vi "终极版程序.vi"() -> ()   [LabVIEW 2013]
uses:
  <vilib>/Platform/TimedLoop/XDataNode/timing_clust.ctl
  <vilib>/Platform/TimedLoop/XDataNode/nitl_modes.ctl
  <vilib>/Platform/TimedLoop/XDataNode/wakeup.ctl
  <vilib>/Simulation/Scripting/Companion Diagram/SimConfigNode/SimParams.ctl
  <vilib>/Simulation/Scripting/Companion Diagram/SimConfigNode/_simSolvers.ctl
  <vilib>/Simulation/Implementation/Shared/SIMSCR Execution Mode.ctl
  <vilib>/Simulation/Param Hierarchy/Typedefs/SIMPH Param Control Actions.ctl
  <vilib>/Simulation/Implementation/Shared/SIM limit type.ctl
  <vilib>/Simulation/Implementation/Shared/NILVSim_ParamChanged.vi
  <vilib>/Simulation/Implementation/Shared/NILVSIM_BeginStep.vi
  <vilib>/Simulation/DataSources/Implementation/NILVSim Signal Generator.llb/SIM Signal Generator (scalar).vi
  <vilib>/Simulation/SignalDisplay/Implementation/NILVSim Time Waveform.llb/SIM Time Waveform (vector).vi
  <vilib>/Simulation/SignalArithmetic/Implementation/NILVSim Gain.llb/SIM Gain (scalar).vi
  <vilib>/Simulation/ContinuousLinear/Implementation/NILVSim Integrator new.llb/SIM Integrator distributor (scalar).vi
  <vilib>/Simulation/Nonlinear/Implementation/NILVSim Saturation.llb/SIM Saturation (scalar).vi
  <vilib>/Simulation/SignalDisplay/Implementation/NILVSim Time Waveform.llb/SIM Time Waveform (scalar).vi
  <vilib>/Simulation/Utility/Implementation/NILVSim Memory.llb/NILVSim Memory (core).vi
  <vilib>/Simulation/ContinuousLinear/Implementation/NILVSim Integrator new.llb/SIM Integrator collector (scalar).vi
  <vilib>/Simulation/Implementation/Shared/NILVSim_Manager.vi
  <vilib>/Simulation/Implementation/Shared/NILVSim_FinalizeModel.vi
  <vilib>/Simulation/Implementation/Shared/SIM Unbundle Sim Info.vi
  <vilib>/Utility/error.llb/Clear Errors.vi
  <vilib>/Simulation/Implementation/Shared/NILVSim_GetModelError.vi
  <vilib>/Simulation/Implementation/Shared/SIM Bundle Sim Info.vi
  <vilib>/Simulation/Implementation/Shared/SIMSH Read Queue.vi
  <vilib>/Simulation/Implementation/Shared/NILVSim_Initialize.vi
  <vilib>/Simulation/Utility/Implementation/NILVSim Get Time and IsAcceptedStep.vi
  <vilib>/Platform/TimedLoop/XDataNode/XDataNode.xnode
  <vilib>/Simulation/Scripting/Companion Diagram/SimConfigNode/SimDog.xnode
  <vilib>/Simulation/Implementation/XNodeFramework/SimXNode/SimX.xnode
  <vilib>/Platform/TimedLoop/XDataNode/XDNodeRunTimeDep.lvlib
  <vilib>/Simulation/ContinuousLinear/Implementation/NILVSim Integrator new.llb/SIM Integrator (scalar).vi
  <vilib>/Simulation/Implementation/Shared/NI_SIM_Implementation.lvlib
panel:
  in  "信号发生器":T1
  out "速度（rad/s）":waveform(dbl)[](graph)
  out "电压（V）":waveform(dbl)(graph)
  in  "PID控制参数":cluster{"kp":dbl, "bsp":dbl, "ki":dbl}
  out "Instrument":string="If you want to exit program,Please press \"Exit Program\" button"
  out "AxMaxVel":bool
  out "DeviceNum List":u32[](array[numeric])
  out "Servo_Off":bool
  in  "Servo_On":bool
  in  "Servo On":bool
  in  "Clear":bool
  out "ChangeV Success":bool
  in  "ChangeV":bool
  in  "Change Velocity":dbl=10000.0
  out "Axis State:":string
  out "CloseSuccess":bool
  in  "Device Type":u16(ring) items=["PCI-1240 (M0)"]
  out "PAR_AxVelHigh":dbl=500.0
  out "Ret_GetCommandPosition":u32
  out "Exit Program":bool
  out "DeviceOpened":bool
  out "AxisOpened":bool
  out "AxisHandle_Array":u32[](array[numeric])
  out "DevAxesCount":u32
  out "EmgSucces":bool
  out "DecSuccess":bool
  in  "Stop Mode":enum32{"Dec", "Emg"}(radio)
  out "RelSucces":bool
  in  "Distance":dbl=50000.0
  out "AbsSuccess":bool
  in  "Movement Mode":enum32{"Absolute", "Relative"}(radio)=enum."Relative"
  in  "Operate Axis":T2(radio)
  in  "Stop":bool
  in  "Move":bool
  out "ResetCounter":bool
  in  "Reset Counter":bool
  out "Axis Position":T3
  out "DeviceHandle":u32
  in  "Stop":bool
  in  "Close Board":bool
  in  "Open Board":bool
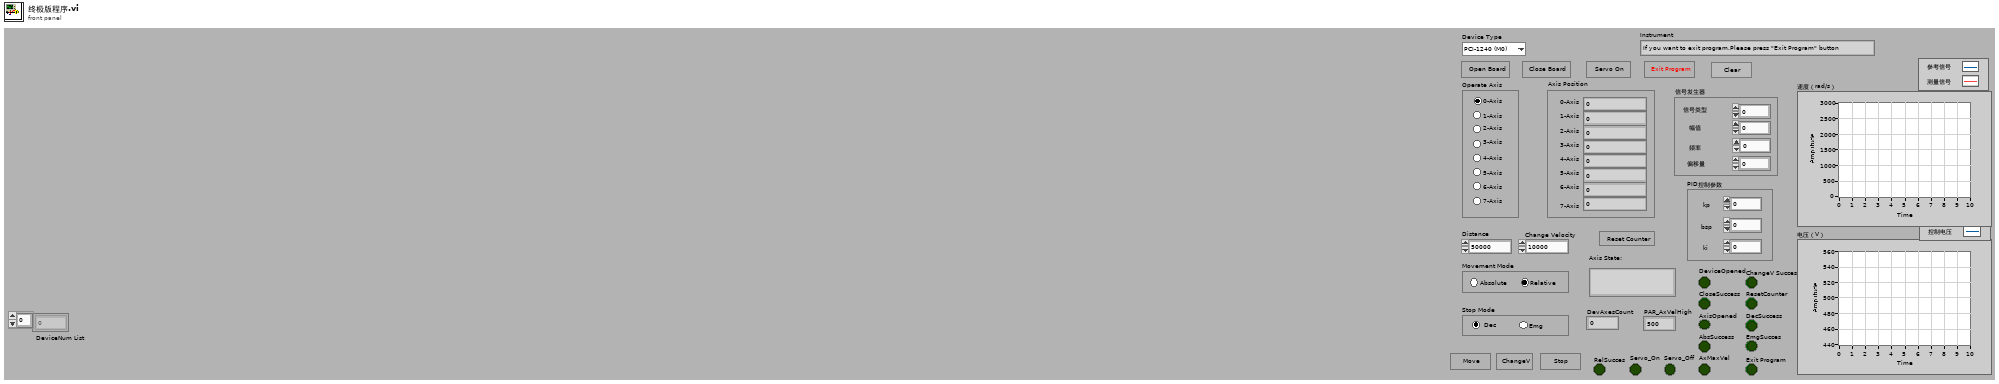
[diagram p1: front panel]
types:
  T1 = cluster{"信号类型":dbl, "幅值":dbl, "频率":dbl, "偏移量":dbl}
  T2 = enum32{"0-Axis", "1-Axis", "2-Axis", "3-Axis", "4-Axis", "5-Axis", "6-Axis", "7-Axis"}
  T3 = cluster{"0-Axis":dbl, "1-Axis":dbl, "2-Axis":dbl, "3-Axis":dbl, "4-Axis":dbl, "5-Axis":dbl, "6-Axis":dbl, "7-Axis":dbl}
  T4 = cluster{"DeviceNum":u32, "U*8 Array":cluster{"U*8 Array[0]":u8, "U*8 Array[1]":u8, "U*8 Array[2]":u8, "U*8 Array[3]":u8, "U*8 Array[4]":u8, "U*8 Array[5]":u8, "U*8 Array[6]":u8, "U*8 Array[7]":u8, "U*8 Array[8]":u8, "U*8 Array[9]":u8, "U*8 Array[10]":u8, "U*8 Array[11]":u8, "U*8 Array[12]":u8, "U*8 Array[13]":u8, "U*8 Array[14]":u8, "U*8 Array[15]":u8, "U*8 Array[16]":u8, "U*8 Array[17]":u8, "U*8 Array[18]":u8, "U*8 Array[19]":u8, "U*8 Array[20]":u8, "U*8 Array[21]":u8, "U*8 Array[22]":u8, "U*8 Array[23]":u8, "U*8 Array[24]":u8, "U*8 Array[25]":u8, "U*8 Array[26]":u8, "U*8 Array[27]":u8, "U*8 Array[28]":u8, "U*8 Array[29]":u8, "U*8 Array[30]":u8, "U*8 Array[31]":u8, "U*8 Array[32]":u8, "U*8 Array[33]":u8, "U*8 Array[34]":u8, "U*8 Array[35]":u8, "U*8 Array[36]":u8, "U*8 Array[37]":u8, "U*8 Array[38]":u8, "U*8 Array[39]":u8, "U*8 Array[40]":u8, "U*8 Array[41]":u8, "U*8 Array[42]":u8, "U*8 Array[43]":u8, "U*8 Array[44]":u8, "U*8 Array[45]":u8, "U*8 Array[46]":u8, "U*8 Array[47]":u8, "U*8 Array[48]":u8, "U*8 Array[49]":u8}, "NumOfSubDevice":i16}[]
  T5 = cluster{"U*8 Array[0]":u8, "U*8 Array[1]":u8, "U*8 Array[2]":u8, "U*8 Array[3]":u8, "U*8 Array[4]":u8, "U*8 Array[5]":u8, "U*8 Array[6]":u8, "U*8 Array[7]":u8, "U*8 Array[8]":u8, "U*8 Array[9]":u8, "U*8 Array[10]":u8, "U*8 Array[11]":u8, "U*8 Array[12]":u8, "U*8 Array[13]":u8, "U*8 Array[14]":u8, "U*8 Array[15]":u8, "U*8 Array[16]":u8, "U*8 Array[17]":u8, "U*8 Array[18]":u8, "U*8 Array[19]":u8, "U*8 Array[20]":u8, "U*8 Array[21]":u8, "U*8 Array[22]":u8, "U*8 Array[23]":u8, "U*8 Array[24]":u8, "U*8 Array[25]":u8, "U*8 Array[26]":u8, "U*8 Array[27]":u8, "U*8 Array[28]":u8, "U*8 Array[29]":u8, "U*8 Array[30]":u8, "U*8 Array[31]":u8, "U*8 Array[32]":u8, "U*8 Array[33]":u8, "U*8 Array[34]":u8, "U*8 Array[35]":u8, "U*8 Array[36]":u8, "U*8 Array[37]":u8, "U*8 Array[38]":u8, "U*8 Array[39]":u8, "U*8 Array[40]":u8, "U*8 Array[41]":u8, "U*8 Array[42]":u8, "U*8 Array[43]":u8, "U*8 Array[44]":u8, "U*8 Array[45]":u8, "U*8 Array[46]":u8, "U*8 Array[47]":u8, "U*8 Array[48]":u8, "U*8 Array[49]":u8}
  T6 = typedef "XDNodeRunTimeDep.lvlib/timing_clust.ctl" = cluster{"Expected End [f-1]":u64, "Actual End [f-1]":u64, "Finished Late? [f-1]":bool, "Expected End [i-1]":u64, "Actual End [i-1]":u64, "Finished Late? [i-1]":bool, "Expected Start [i]":u64, "Actual Start [i]":u64, "Expected Start [f]":u64, "Actual Start [f]":u64, "Source Name":string, "Structure Name":string, "Period":i64, "Deadline":i64, "Offset":i64, "Start":i64, "Priority":i32, "Timeout":i32, "Mode":T7, "Wakeup Reason":T8, "Error":errorcluster, "Source Type":string, "Secondary Source Type":string, "Global End Time":u64, "Global Start Time":u64, "Frame Duration":u64, "Iteration Duration":u64, "Assigned CPU":i32, "I/O Scan Engine Mode":u32}
  T7 = typedef "XDNodeRunTimeDep.lvlib/nitl_modes.ctl" = enum32{"No Change", "Process missed periods, maintain original phase", "Discard missed periods, maintain original phase", "Process missed periods, ignore original phase", "Discard missed periods, ignore original phase"}
  T8 = typedef "XDNodeRunTimeDep.lvlib/wakeup.ctl" = enum32{"Normal", "Aborted", "Asynchronous wakeup", "Timing source error", "Timed loop error", "Timeout"}
  T9 = typedef "SIMSCR Execution Mode.ctl" = enum16{"Simulate to Completion", "Single Time-Step Simulation (Fixed Step Only)"}
  T10 = typedef "SIMPH Param Control Actions.ctl" = enum16{"get params", "set params"}
  T11 = typedef "SIM limit type.ctl" = enum16{"upper", "lower", "both", "none"}
  T12 = typedef "SimParams.ctl" = cluster{"Initial Time (s)":dbl, "Final Time (s)":dbl, "Step Size (s)":dbl, "ODE Solver":T13, "Minimum Step Size (s)":dbl, "Maximum Step Size (s)":dbl, "Relative Tolerance":dbl, "Absolute Tolerance":dbl, "Software Timing":bool, "Initial Step Size (s)":dbl, "Automatic Fixed Step Size?":bool, "Automatic Discrete Step Size?":bool, "Discrete Step Size (s)":dbl, "Calculate using Time Step":bool, "Solver Wired?":bool, "Prev.Frm.Expected End":u64, "Prev.Frm.Actual End":u64, "Prev.Frm.Finished Late?":bool, "Prev.Iter.Expected End":u64, "Prev.Iter.Actual End":u64, "Prev.Iter.Finished Late?":bool, "Expected Iteration Start":u64, "Actual Iteration Start":u64, "Expected Frame Start":u64, "Actual Frame Start":u64, "Source Name":string, "Name":string, "Period":i64, "Deadline":i64, "Offset":i64, "Start":i64, "Priority":i32, "Timeout":i32, "Processor":i32, "Mode":enum32{"No Change", "Process missed periods, maintain original phase", "Discard missed periods, maintain original phase", "Process missed periods, ignore original phase", "Discard missed periods, ignore original phase"}, "Wakeup reason":enum32{"Normal", "Aborted", "Asynchronous wakeup", "Timing source error", "Timed loop error", "Timeout"}, "Error":errorcluster, "Source Type":string, "Secondary Source Type":string, "Global End Time":u64, "Global Start Time":u64, "Full Solver Reset":bool, "Execution Mode":T9, "Nan/Inf Check":bool, "Custom Solver Library":string, "Solver Is Variable":bool, "custom solver name":string, "Signal Collection Decimation":u32}
  T13 = typedef "_simSolvers.ctl" = enum16{"Runge-Kutta 1 (Euler)", "Runge-Kutta 2", "Runge-Kutta 3", "Runge-Kutta 4", "Runge-Kutta 23 (variable)", "Runge-Kutta 45 (variable)", "BDF (variable)", "Adams-Moulton (variable)", "Rosenbrock (variable)", "Discrete States Only", "SDIRK 4 (variable)", "Radau 5 (variable)", "Radau 9 (variable)", "Radau 13 (variable)", "Radau [Variable Order] (variable)", "Gear's Method (variable)", "Linearizer", "State Query", "Trim Eval", "Custom Solver"}
  T14 = cluster{"[0]":dbl, "[1]":dbl, "[2]":dbl, "[3]":dbl, "[4]":dbl, "[5]":dbl, "[6]":dbl, "[7]":dbl}
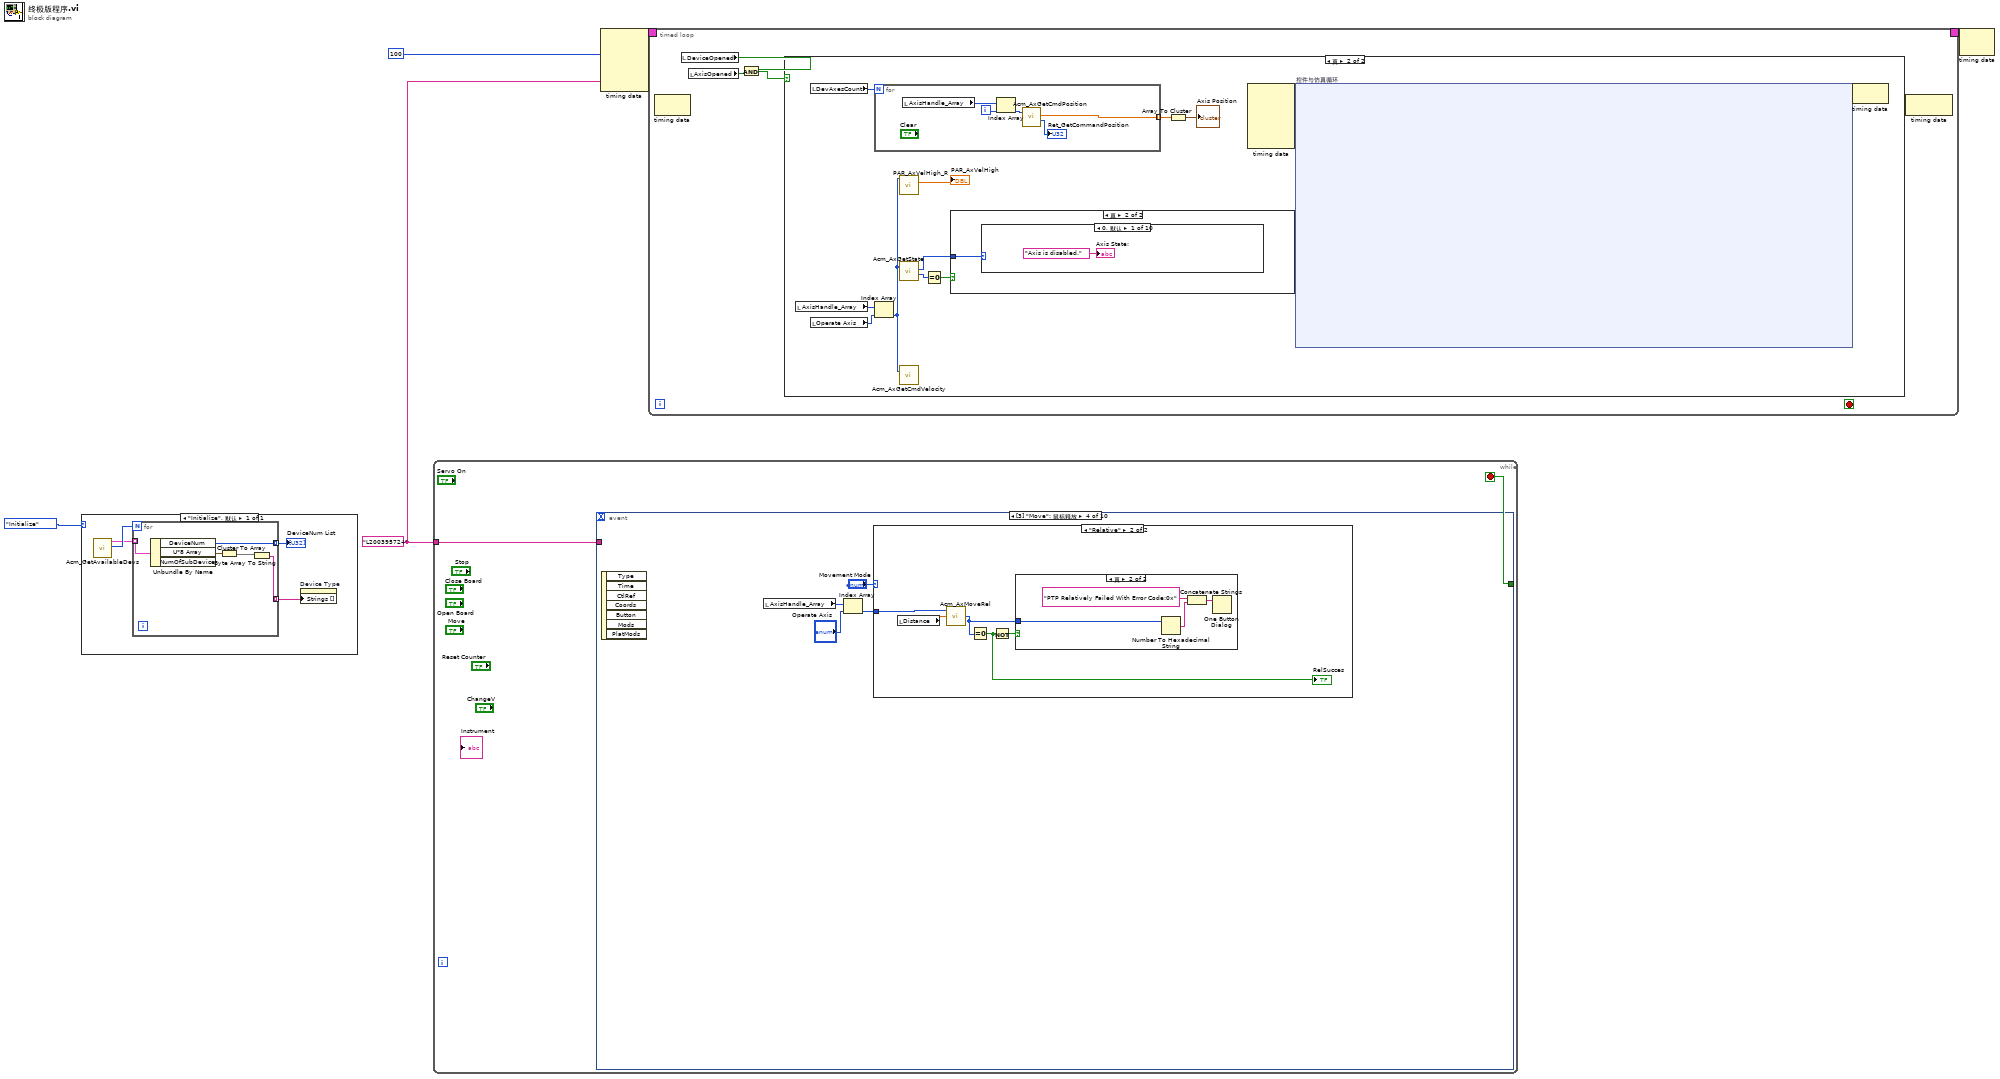
[diagram p0: block diagram]
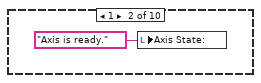
[diagram p4: hidden frame]
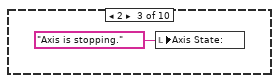
[diagram p5: hidden frame]
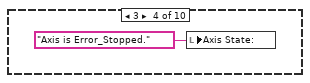
[diagram p6: hidden frame]
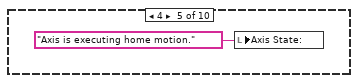
[diagram p7: hidden frame]
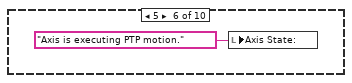
[diagram p8: hidden frame]
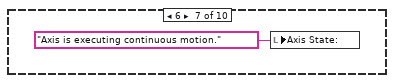
[diagram p9: hidden frame]
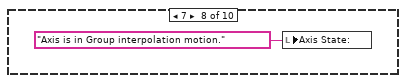
[diagram p10: hidden frame]
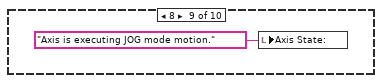
[diagram p11: hidden frame]
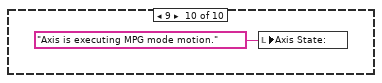
[diagram p12: hidden frame]
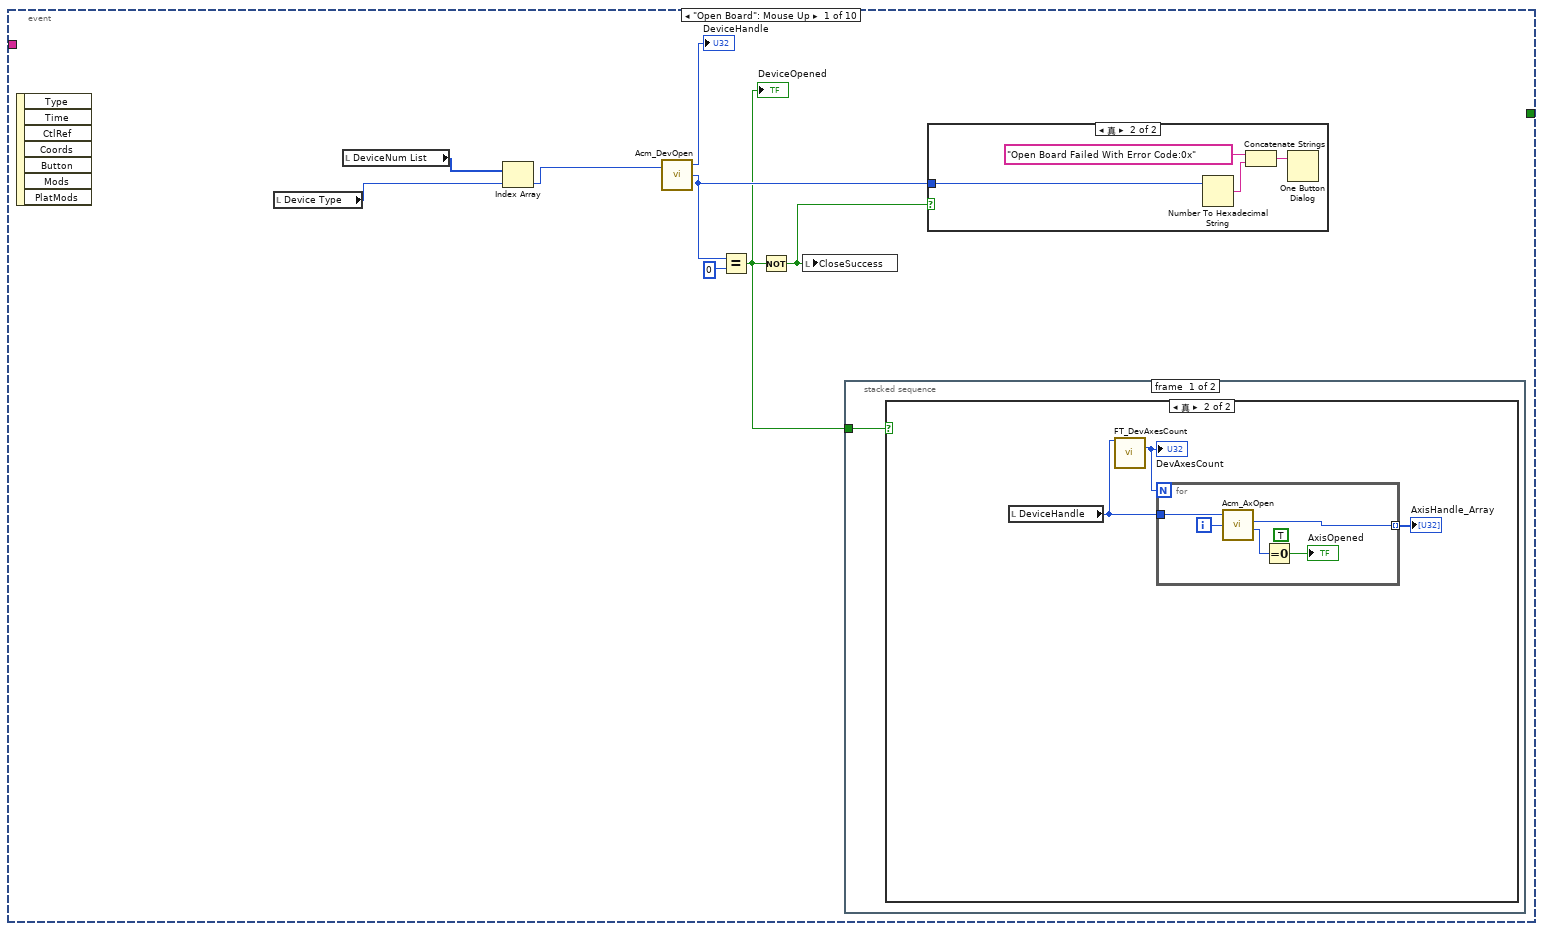
[diagram p13: hidden frame]
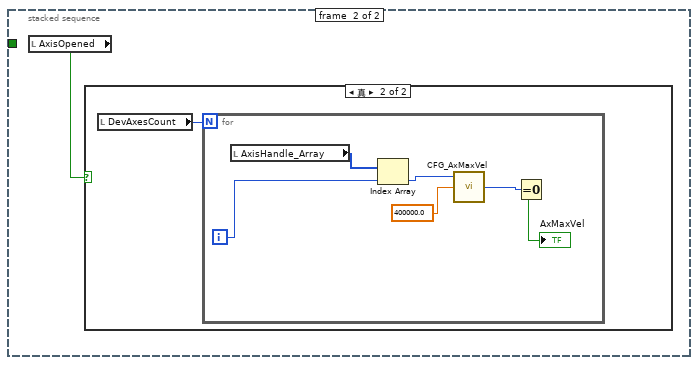
[diagram p15: hidden frame]
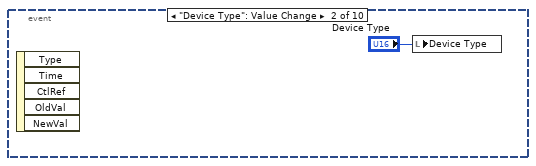
[diagram p18: hidden frame]
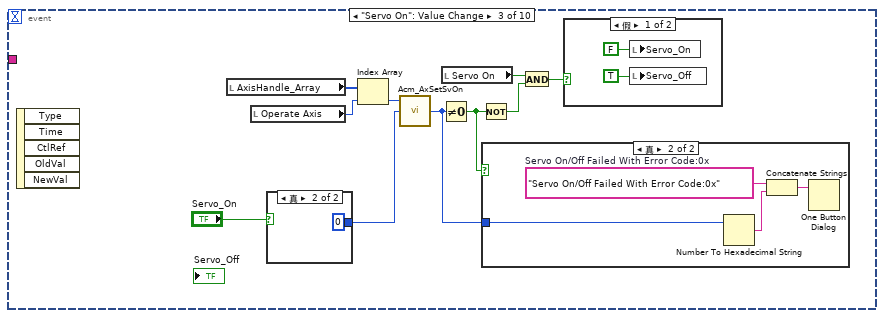
[diagram p19: hidden frame]
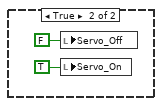
[diagram p20: hidden frame]
diagram:
  w2 = "L200395724" ("结构名称")
  n1 = case shown="\"Initialize\", 默认" enum16{"Initialize"}."Initialize" ("Enum") {
    frame "Initialize", Default {
      n2 = call <userlib>:"Acm_GetAvailableDevs.vi"() -> ("DeviceList"=w8:T4, "OutEntries"=w9:u32)  [unwired: 1 in, 4 out]
      n3 = for {
        N: w9 -> [_]
        tunnel: w8 -> [w14] mode=indexing
        tunnel: [w11] -> w7 mode=indexing
        tunnel: [w10] -> w6 mode=indexing
        n4 = Unbundle By Name(w14) -> ("DeviceNum"=w11:u32, "U*8 Array"=w13:T5)  [unwired: 1 out]
        n5 = Cluster To Array(cluster=w13) -> (array=w12:u8[])
        n6 = Byte Array To String(unsigned byte array=w12) -> (string=w10:string)
      }
      "DeviceNum List" <- w7
      n7 = property on="Device Type" class="Ring (严格)"("Strings []"=w6) -> ()  [unwired: 2 in, 2 out]
    }
  }
  n8 = while {
    tunnel: w2 -> [w16]
    stop <- w15 stop-if-true
    n9 = event shown="[3] \"Move\": 鼠标释放" {
      selector: _ -> [_ _ _ _ _ _ _ _ _ _]
      dyn-events: _ -> [_ _ _ _ _ _ _ _ _ _]
      timeout: _ -> [_ _ _ _ _ _ _ _ _ _]
      tunnel: w16 -> [_ _ _ _ _ _ _ _ _ w151]
      tunnel: [_ _ _ _ _ _ _ _ _ "Stop"] -> w15
      event "Open Board": Mouse Up {
        n10 = event-data() -> ()  [unwired: 8 out]
        n11 = local read "Device Type"() -> (w18:u16)
        n12 = local read "DeviceNum List"() -> (w20:u32[])
        n13 = Index Array(array=w20, index=w18) -> (element=w19:u32)
        n14 = call <userlib>:"Acm_DevOpen.vi"("DeviceNumber"=w19) -> ("ReturnValue"=w22:u32, "DeviceHandle"=→"DeviceHandle":u32)  [unwired: 1 in, 1 out]
        n15 = Equal?(x=w22, y=u32 0) -> (x = y?=w17:bool)
        "DeviceOpened" <- w17
        n16 = Not(x=w17) -> (.not. x?=w21:bool)
        n17 = local write "CloseSuccess"(w21) -> ()
        n18 = stacked-sequence {
          tunnel: w17 -> [w25 _]
          frame #0 {
            n19 = case shown="真" w25 {
              frame False {
              }
              frame True {
                n20 = local read "DeviceHandle"() -> (w27:u32)
                n21 = call <userlib>:"FT_DevAxesCount.vi"("Handle"=w27) -> ("DevAxesCount"=w28:u32)  [unwired: 1 in, 13 out]
                "DevAxesCount" <- w28
                n22 = for {
                  N: w28 -> [_]
                  tunnel: w27 -> [w33]
                  tunnel: [w29] -> w26 mode=indexing
                  i -> [w32]
                  (unwired) TRUE ("AxisOpened")
                  n23 = call <userlib>:"Acm_AxOpen.vi"("PhyAxis"=w32, "DeviceHandle"=w33) -> ("ReturnValue"=w31:u32, "AxisHandle"=w29:u32)  [unwired: 1 in, 2 out]
                  n24 = Equal To 0?(x=w31) -> (x = 0?=→"AxisOpened":bool)
                }
                "AxisHandle_Array" <- w26
              }
            }
          }
          frame #1 {
            n25 = local read "AxisOpened"() -> (w34:bool)
            n26 = case shown="真" w34 {
              frame False {
              }
              frame True {
                n27 = local read "DevAxesCount"() -> (w35:u32)
                n28 = for {
                  N: w35 -> [_]
                  i -> [w37]
                  n29 = local read "AxisHandle_Array"() -> (w38:u32[])
                  n30 = Index Array(array=w38, index=w37) -> (element=w39:u32)
                  n31 = call <userlib>:"CFG_AxMaxVel.vi"("CFG_AxMaxVel"=400000.0, "Handle"=w39) -> ("ReturnValue"=w41:u32)  [unwired: 1 in, 2 out]
                  n32 = Equal To 0?(x=w41) -> (x = 0?=→"AxMaxVel":bool)
                }
              }
            }
          }
        }
        n33 = case shown="真" w21 {
          tunnel: w22 -> [_ w45]
          frame False {
          }
          frame True {
            n34 = Number To Hexadecimal String(2:w45) -> (0:w43:string)  [unwired: 1 out]
            n35 = Concatenate Strings("Open Board Failed With Error Code:0x", w43) -> (w42:string)
            n36 = One Button Dialog(message=w42) -> ()  [unwired: 2 out]
          }
        }
      }
      event "Device Type": Value Change {
        n37 = event-data() -> ()  [unwired: 6 out]
        n38 = local write "Device Type"("Device Type") -> ()
      }
      event "Servo On": Value Change {
        n39 = event-data() -> ()  [unwired: 6 out]
        n40 = local read "AxisHandle_Array"() -> (w56:u32[])
        n41 = local read "Operate Axis"() -> (w55:T2)
        n42 = case shown="真" "Servo_On" {
          tunnel: [u32 1 u32 0] -> w53
          frame False {
          }
          frame True {
          }
        }
        n43 = Index Array(array=w56, index=w55) -> (element=w54:u32)
        n44 = call <userlib>:"Acm_AxSetSvOn.vi"("OnOff"=w53, "AxisHandle"=w54) -> ("ReturnValue"=w47:u32)  [unwired: 1 in, 2 out]
        n45 = Not Equal To 0?(x=w47) -> (x != 0?=w52:bool)
        n46 = local read "Servo On"() -> (w50:bool)
        n47 = Not(x=w52) -> (.not. x?=w51:bool)
        n48 = case shown="真" w52 {
          tunnel: w47 -> [_ w61]
          frame False {
          }
          frame True {
            w64 = "Servo On/Off Failed With Error Code:0x"  # Servo On/Off Failed With Error Code:0x
            n49 = Number To Hexadecimal String(2:w61) -> (0:w63:string)  [unwired: 1 out]
            n50 = Concatenate Strings(w64, w63) -> (w62:string)
            n51 = One Button Dialog(message=w62) -> ()  [unwired: 2 out]
          }
        }
        n52 = And(x=w50, y=w51) -> (x .and. y?=w49:bool)
        n53 = case shown="假" w49 {
          frame False {
            n54 = local write "Servo_On"(FALSE ("Servo_On")) -> ()
            n55 = local write "Servo_Off"(TRUE ("Servo_Off")) -> ()
          }
          frame True {
            n56 = local write "Servo_Off"(FALSE ("Servo_Off")) -> ()
            n57 = local write "Servo_On"(TRUE ("Servo_On")) -> ()
          }
        }
      }
      event "Move": Mouse Up {
        n58 = event-data() -> ()  [unwired: 8 out]
        n59 = local read "AxisHandle_Array"() -> (w70:u32[])
        n60 = Index Array(array=w70, index="Operate Axis") -> (element=w69:u32)
        n61 = case shown="\"Relative\"" "Movement Mode" {
          tunnel: w69 -> [w75 w84]
          frame "Absolute", Default {
            n62 = call <userlib>:"Acm_AxMoveAbs.vi"("Position"="Distance", "AxisHandle"=w75) -> ("ReturnValue"=w73:u32)  [unwired: 1 in, 2 out]
            n63 = Equal To 0?(x=w73) -> (x = 0?=w72:bool)
            "AbsSuccess" <- w72
            n64 = Not(x=w72) -> (.not. x?=w71:bool)
            n65 = case shown="真" w71 {
              tunnel: w73 -> [_ w76]
              frame False {
              }
              frame True {
                n66 = Number To Hexadecimal String(2:w76) -> (0:w78:string)  [unwired: 1 out]
                n67 = Concatenate Strings("PTP Absolutely failed with Error Code:0x", w78) -> (w77:string)
                n68 = One Button Dialog(message=w77) -> ()  [unwired: 2 out]
              }
            }
          }
          frame "Relative" {
            n69 = local read "Distance"() -> (w83:dbl)
            n70 = call <userlib>:"Acm_AxMoveRel.vi"("Distance"=w83, "AxisHandle"=w84) -> ("ReturnValue"=w82:u32)  [unwired: 1 in, 2 out]
            n71 = Equal To 0?(x=w82) -> (x = 0?=w80:bool)
            "RelSucces" <- w80
            n72 = Not(x=w80) -> (.not. x?=w81:bool)
            n73 = case shown="真" w81 {
              tunnel: w82 -> [_ w85]
              frame False {
              }
              frame True {
                n74 = Number To Hexadecimal String(2:w85) -> (0:w87:string)  [unwired: 1 out]
                n75 = Concatenate Strings("PTP Relatively Failed With Error Code:0x", w87) -> (w86:string)
                n76 = One Button Dialog(message=w86) -> ()  [unwired: 2 out]
              }
            }
          }
        }
      }
      event "ChangeV": Mouse Up {
        n77 = event-data() -> ()  [unwired: 8 out]
        n78 = local read "AxisHandle_Array"() -> (w95:u32[])
        n79 = local read "Operate Axis"() -> (w94:T2)
        n80 = Index Array(array=w95, index=w94) -> (element=w93:u32)
        n81 = call <userlib>:"Acm_AxChangeVel.vi"("NewVelocity"="Change Velocity", "AxisHandle"=w93) -> ("ReturnValue"=w91:u32)  [unwired: 1 in, 2 out]
        n82 = Equal To 0?(x=w91) -> (x = 0?=w89:bool)
        "ChangeV Success" <- w89
        n83 = Not(x=w89) -> (.not. x?=w90:bool)
        n84 = case shown="真" w90 {
          tunnel: w91 -> [_ w96]
          frame False {
          }
          frame True {
            n85 = Number To Hexadecimal String(2:w96) -> (0:w98:string)  [unwired: 1 out]
            n86 = Concatenate Strings("Change Velocity Failed With Error Code:0x", w98) -> (w97:string)
            n87 = One Button Dialog(message=w97) -> ()  [unwired: 2 out]
          }
        }
      }
      event "Stop": Mouse Up {
        n88 = event-data() -> ()  [unwired: 8 out]
        n89 = local read "AxisHandle_Array"() -> (w103:u32[])
        n90 = local read "Operate Axis"() -> (w101:T2)
        n91 = Index Array(array=w103, index=w101) -> (element=w102:u32)
        n92 = case shown="\"Dec\", 默认" "Stop Mode" {
          tunnel: w102 -> [w107 w114]
          frame "Dec", Default {
            n93 = call <userlib>:"Acm_AxStopDec.vi"("AxisHandle"=w107) -> ("ReturnValue"=w105:u32)  [unwired: 1 in, 2 out]
            n94 = Equal To 0?(x=w105) -> (x = 0?=w104:bool)
            "DecSuccess" <- w104
            n95 = Not(x=w104) -> (.not. x?=w106:bool)
            n96 = case shown="真" w106 {
              tunnel: w105 -> [_ w111]
              frame False {
              }
              frame True {
                n97 = Number To Hexadecimal String(2:w111) -> (0:w109:string)  [unwired: 1 out]
                n98 = Concatenate Strings("Stop Failed With Error Code:0x", w109) -> (w108:string)
                n99 = One Button Dialog(message=w108) -> ()  [unwired: 2 out]
              }
            }
          }
          frame "Emg" {
            n100 = call <userlib>:"Acm_AxStopEmg.vi"("AxisHandle"=w114) -> ("ReturnValue"=w112:u32)  [unwired: 1 in, 2 out]
            n101 = Equal To 0?(x=w112) -> (x = 0?=w113:bool)
            "EmgSucces" <- w113
            n102 = Not(x=w113) -> (.not. x?=w115:bool)
            n103 = case shown="真" w115 {
              tunnel: w112 -> [_ w119]
              frame False {
              }
              frame True {
                n104 = Number To Hexadecimal String(2:w119) -> (0:w117:string)  [unwired: 1 out]
                n105 = Concatenate Strings("Stop failed with Error Code:0x", w117) -> (w116:string)
                n106 = One Button Dialog(message=w116) -> ()  [unwired: 2 out]
              }
            }
          }
        }
      }
      event "Clear": Mouse Up {
        n107 = event-data() -> ()  [unwired: 8 out]
      }
      event "Reset Counter": Mouse Up {
        n108 = event-data() -> ()  [unwired: 8 out]
        n109 = local read "AxisOpened"() -> (w120:bool)
        n110 = case shown="真" w120 {
          frame False {
          }
          frame True {
            n111 = local read "DevAxesCount"() -> (w121:u32)
            n112 = for {
              N: w121 -> [_]
              i -> [w126]
              n113 = local read "AxisHandle_Array"() -> (w127:u32[])
              n114 = Index Array(array=w127, index=w126) -> (element=w125:u32)
              n115 = call <userlib>:"Acm_AxSetCmdPosition.vi"("Position"=0.0, "AxisHandle"=w125) -> ("ReturnValue"=w123:u32)  [unwired: 1 in, 2 out]
              n116 = Equal To 0?(x=w123) -> (x = 0?=→"ResetCounter":bool)
            }
          }
        }
      }
      event "Close Board": Mouse Up {
        n117 = event-data() -> ()  [unwired: 8 out]
        n118 = stacked-sequence {
          frame #0 {
            n119 = local read "DevAxesCount"() -> (w128:u32)
            n120 = for {
              N: w128 -> [_]
              i -> [w133]
              n121 = local read "AxisHandle_Array"() -> (w134:u32[])
              n122 = Index Array(array=w134, index=w133) -> (element=w132:u32)
              n123 = call <userlib>:"Acm_AxClose.vi"("AxisHandle"=w132) -> ("ReturnValue"=w131:u32)  [unwired: 1 in, 1 out]
              n124 = Equal To 0?(x=w131) -> (x = 0?=w130:bool)
              n125 = Not(x=w130) -> (.not. x?=w129:bool)
              n126 = local write "AxisOpened"(w129) -> ()
            }
          }
          frame #1 {
            n127 = local read "DeviceHandle"() -> (w138:u32)
            n128 = call <userlib>:"Acm_DevClose.vi"("DeviceHandle"=w138) -> ("ReturnValue"=w136:u32)  [unwired: 1 in, 3 out]
            n129 = Equal To 0?(x=w136) -> (x = 0?=w135:bool)
            "CloseSuccess" <- w135
            n130 = Not(x=w135) -> (.not. x?=w137:bool)
            n131 = case shown="真" w135 {
              tunnel: w135 -> [_ w144]
              frame False {
              }
              frame True {
                n132 = Not(x=w144) -> (.not. x?=w143:bool)
                n133 = local write "DevAxesCount"(u32 0 ("DevAxesCount")) -> ()
                n134 = local write "DeviceHandle"(u32 0 ("DeviceHandle")) -> ()
                n135 = local write "ChangeV Success"(w143) -> ()
                n136 = local write "DeviceOpened"(w143) -> ()
                n137 = local write "RelSucces"(w143) -> ()
                n138 = local write "DecSuccess"(w143) -> ()
                n139 = local write "ResetCounter"(w143) -> ()
                n140 = local write "AbsSuccess"(w143) -> ()
                n141 = local write "EmgSucces"(w143) -> ()
                n142 = local read "DevAxesCount"() -> (w147:u32)
                n143 = Initialize Array(u32 0 ("元素"), w147) -> (w146:u32[])
                n144 = local write "AxisHandle_Array"(w146) -> ()
              }
            }
            n145 = case shown="真" w137 {
              tunnel: w136 -> [_ w142]
              frame False {
              }
              frame True {
                n146 = Number To Hexadecimal String(2:w142) -> (0:w140:string)  [unwired: 1 out]
                n147 = Concatenate Strings("Close Board Failed With Error Code:0x", w140) -> (w139:string)
                n148 = One Button Dialog(message=w139) -> ()  [unwired: 2 out]
              }
            }
          }
        }
      }
      event "Stop": Value Change {
        n149 = event-data() -> ()  [unwired: 6 out]
        n150 = call <vilib>:"Stop Timed Structure.vi"("name"=w151) -> ()  [unwired: 2 in, 9 out]
        "Exit Program" <- "Stop"
      }
    }
  }
  n151 = node-c288(i64 100 ("周期"), w2) -> (w5:T6)  [unwired: 3 out]
  n152 = timed-loop {
    timing: w5 -> [_]
    timing-out: [_] -> w4
    stop <- _ stop-if-true
    n153 = node-c288() -> ()  [unwired: 2 out]
    n154 = local read "DeviceOpened"() -> (w154:bool)
    n155 = local read "AxisOpened"() -> (w153:bool)
    n156 = And(x=w154, y=w153) -> (x .and. y?=w152:bool)
    n157 = case shown="真" w152 {
      frame False {
      }
      frame True {
        n158 = local read "AxisHandle_Array"() -> (w163:u32[])
        n159 = local read "DevAxesCount"() -> (w164:u32)
        n160 = local read "Operate Axis"() -> (w162:T2)
        n161 = for {
          N: w164 -> [_]
          tunnel: [w692] -> w165 mode=indexing
          i -> [w694]
          n162 = local read "AxisHandle_Array"() -> (w695:u32[])
          n163 = Index Array(array=w695, index=w694) -> (element=w693:u32)
          n164 = call <userlib>:"Acm_AxGetCmdPosition.vi"("AxisHandle"=w693) -> ("ReturnValue"=→"Ret_GetCommandPosition":u32, "Position"=w692:dbl)  [unwired: 1 in, 2 out]
        }
        n165 = Index Array(array=w163, index=w162) -> (element=w158:u32)
        n166 = call <userlib>:"PAR_AxVelHigh_R.vi"("Handle"=w158) -> ("PAR_AxVelHigh"=→"PAR_AxVelHigh":dbl)  [unwired: 1 in, 13 out]
        n167 = call <userlib>:"Acm_AxGetState.vi"("AxisHandle"=w158) -> ("ReturnValue"=w161:u32, "Status"=w159:u16)  [unwired: 1 in, 2 out]
        n168 = call <userlib>:"Acm_AxGetCmdVelocity.vi"("AxisHandle"=w158) -> ()  [unwired: 1 in, 4 out]
        n169 = Equal To 0?(x=w161) -> (x = 0?=w160:bool)
        n170 = case shown="真" w160 {
          tunnel: w159 -> [_ w680]
          frame False {
          }
          frame True {
            n171 = case shown="0, 默认" w680 {
              frame 0, Default {
                "Axis State:" <- "Axis is disabled." ("Axis State:")
              }
              frame 1 {
                n172 = local write "Axis State:"("Axis is ready." ("Axis State:")) -> ()
              }
              frame 2 {
                n173 = local write "Axis State:"("Axis is stopping." ("Axis State:")) -> ()
              }
              frame 3 {
                n174 = local write "Axis State:"("Axis is Error_Stopped." ("Axis State:")) -> ()
              }
              frame 4 {
                n175 = local write "Axis State:"("Axis is executing home motion." ("Axis State:")) -> ()
              }
              frame 5 {
                n176 = local write "Axis State:"("Axis is executing PTP motion." ("Axis State:")) -> ()
              }
              frame 6 {
                n177 = local write "Axis State:"("Axis is executing continuous motion." ("Axis State:")) -> ()
              }
              frame 7 {
                n178 = local write "Axis State:"("Axis is in Group interpolation motion." ("Axis State:")) -> ()
              }
              frame 8 {
                n179 = local write "Axis State:"("Axis is executing JOG mode motion." ("Axis State:")) -> ()
              }
              frame 9 {
                n180 = local write "Axis State:"("Axis is executing MPG mode motion." ("Axis State:")) -> ()
              }
            }
          }
        }
        n181 = Array To Cluster(array=w165) -> (cluster=→"Axis Position":T14)
        n182 = node-c288() -> (w156:variant)  [unwired: 6 in]
        n183 = node-c254 "控件与仿真循环"(w156) -> (w155:variant)
        n184 = node-c288(w155) -> ()  [unwired: 1 out]
      }
    }
    n185 = node-c288() -> ()  [unwired: 2 out]
  }
  n186 = node-c288(w4) -> ()  [unwired: 1 out]
